vi "Volts_to_temperature_(SubVI).vi"(4 "ch_data_string":string, 7 "error in":errorcluster, 16 "koeff. cluster":T1 {"k7" format="%#_18g"; "k6" format="%#_18g"; "k5" format="%#_18g"; "k4" format="%#_18g"; "k3" format="%#_18g"; "k2" format="%#_18g"; "k1" format="%#_18g"}) -> (9 "s? color":u32, 10 "Vin < 0?":bool, 20 "T solvation":dbl, 21 "meas_voltage":dbl, 27 "error out":errorcluster)   [LabVIEW 2015]
uses:
  <vilib>/express/express arith-compare/Formula/XNode/ExpressFormulaBlockNode.xnode
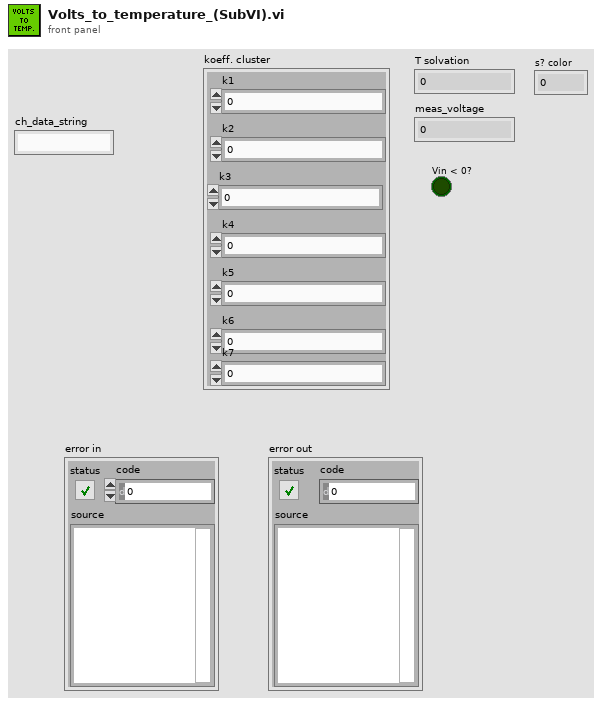
[diagram p1: front panel]
types:
  T1 = cluster{"k1":ext, "k2":ext, "k3":ext, "k4":ext, "k5":ext, "k6":ext, "k7":ext}
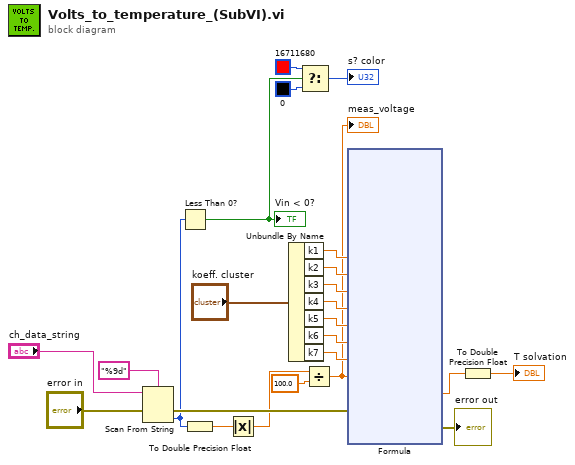
[diagram p0: block diagram]
diagram:
  n1 = Scan From String(format string="%9d", input string="ch_data_string", error in="error in") -> (error out=w9:errorcluster, output 1=w7:i32)  [unwired: 2 in, 2 out]
  n2 = Less Than 0?(x=w7) -> (x < 0?=w19:bool)
  "Vin < 0?" <- w19
  n3 = To Double Precision Float(number=w7) -> (double precision float=w17:dbl)
  n4 = Absolute Value(x=w17) -> (abs(x)=w4:dbl)
  n5 = Unbundle By Name("koeff. cluster") -> ("k1"=w16:ext, "k2"=w15:ext, "k3"=w14:ext, "k4"=w13:ext, "k5"=w12:ext, "k6"=w11:ext, "k7"=w10:ext)
  n6 = Select(t=u32 16711680, s=w19, f=u32 0) -> (s? t:f=→"s? color":u32)
  n7 = Divide(x=w4, y=100.0) -> (x/y=w6:dbl)
  "meas_voltage" <- w6
  n8 = xnode "Formula"("k1"=w16, "k2"=w15, "k3"=w14, "k4"=w13, "k5"=w12, "k6"=w11, "k7"=w10, "Rin"=w6, "error in (no error)"=w9) -> ("Result"=w2:ext, "error out"=→"error out":errorcluster)
  n9 = To Double Precision Float(number=w2) -> (double precision float=→"T solvation":dbl)
